vi "xiLIB - GPIO_Editor.vi"(8 "error in (no error)":errorcluster, 11 "xiCam In":refnum<k24>) -> (0 "error out":errorcluster)   [LabVIEW 2018]
doc: "Dialog based GPIO editor."
uses:
  xiCam/PRM/GPI_MODE/GPI_MODE.ctl
  xiCam/PRM/GPO_MODE/GPO_MODE.ctl
  D:/codes labview/VisionLibrariesXimea/xiLib/xiLIB_64bit/xiLIB/xiCamLib/API/x64/xiApi.NETX64.dll
  API/x64/xiApi.NETX64.dll
  xiCam/PRM/PRM/PRM_v2.ctl
panel:
  in  "GPO_MODE":T1
  in  "GPO_SELECTOR":u16(ring) items=["GPO 1"=1]
  in  "GPI_MODE":T2
  in  "GPI_SELECTOR":u16(ring) items=["GPI 1"=1]
  # "GPI/O Settings"
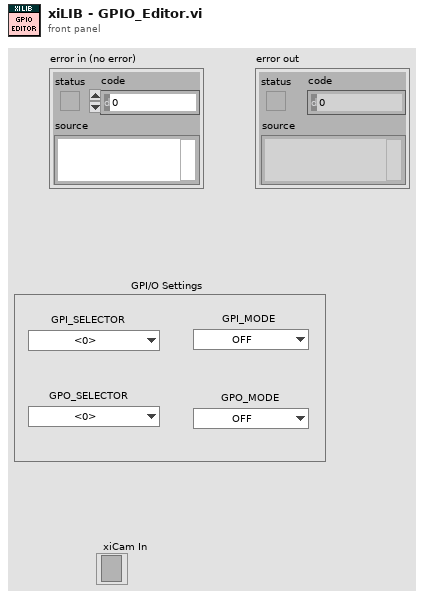
[diagram p1: front panel]
types:
  T1 = typedef "GPO_MODE.ctl" = enum16{"OFF", "ON", "FRAME_ACTIVE", "FRAME_ACTIVE_NEG", "EXPOSURE_ACTIVE", "EXPOSURE_ACTIVE_NEG"}
  T2 = typedef "GPI_MODE.ctl" = enum16{"OFF", "TRIGGER", "EXT_EVENT"}
  T3 = typedef "PRM_v2.ctl" = enum16{"ACQ_BUFFER_SIZE", "ACQ_FRAME_BURST_COUNT", "ACQ_TIMING_MODE", "ACQ_TRANSPORT_BUFFER_SIZE", "AE_MAX_LIMIT", "AEAG", "AEAG_LEVEL", "API_VERSION", "AG_MAX_LIMIT", "APPLY_CMS", "AUTO_BANDWIDTH_CALCULATION", "AUTO_WB", "AVAILABLE_BANDWIDTH", "AVAILABLE_BANDWIDTH_MAX", "AVAILABLE_BANDWIDTH_MIN", "BPC", "BUFFER_POLICY", "BUFFERS_QUEUE_SIZE", "CC_MATRIX_00", "CC_MATRIX_01", "CC_MATRIX_02", "CC_MATRIX_03", "CC_MATRIX_10", "CC_MATRIX_11", "CC_MATRIX_12", "CC_MATRIX_13", "CC_MATRIX_20", "CC_MATRIX_21", "CC_MATRIX_22", "CC_MATRIX_23", "CC_MATRIX_30", "CC_MATRIX_31", "CC_MATRIX_32", "CC_MATRIX_33", "CHIP_TEMP", "CMS", "COLOR_FILTER_ARRAY", "COOLING", "DEBOUNCE_EN", "DEBOUNCE_POL", "DEBOUNCE_T0", "DEBOUNCE_T1", "DEBUG_LEVEL", "DEFAULT_CC_MATRIX", "DEVICE_INSTANCE_PATH", "DEVICE_MODEL_ID", "DEVICE_NAME", "DEVICE_SN", "DEVICE_TYPE", "DEVICE_USER_ID", "DOWNSAMPLING", "DOWNSAMPLING_MAX", "DOWNSAMPLING_MIN", "DOWNSAMPLING_TYPE", "DRV_VERSION", "EXP_PRIORITY", "EXPOSURE", "EXPOSURE_DIRECT_UPDATE", "EXPOSURE_MAX", "EXPOSURE_MIN", "FFS_FILE_NAME", "FPGA1_VERSION", "FRAMERATE", "FRAMERATE_MAX", "FRAMERATE_MIN", "FREE_FFS_SIZE", "GAIN", "GAIN_DIRECT_UPDATE", "GAIN_MAX", "GAIN_MIN", "GAMMAC", "GAMMAY", "GPI_LEVEL", "GPI_MODE", "GPI_SELECTOR", "GPI_SELECTOR_MAX", "GPI_SELECTOR_MIN", "GPO_MODE", "GPO_SELECTOR", "GPO_SELECTOR_MAX", "GPO_SELECTOR_MIN", "HDR", "HDR_T1", "HDR_T2", "HEIGHT", "HEIGHT_MAX", "HEIGHT_MIN", "HOUSE_TEMP", "IMAGE_DATA_FORMAT", "IMAGE_IS_COLOR", "INPUT_CMS_PROFILE", "IS_COOLED", "IS_DEVICE_EXIST", "KNEEPOINT1", "KNEEPOINT2", "LED_MODE", "LED_SELECTOR", "LED_SELECTOR_MAX", "LED_SELECTOR_MIN", "LIMIT_BANDWIDTH", "LIMIT_BANDWIDTH_MAX", "LIMIT_BANDWIDTH_MIN", "LUT_EN", "LUT_INDEX", "LUT_INDEX_MAX", "LUT_INDEX_MIN", "LUT_VALUE", "LUT_VALUE_MAX", "LUT_VALUE_MIN", "MANUAL_WB", "MCU1_VERSION", "MCU2_VERSION", "OFFSET_X", "OFFSET_X_MAX", "OFFSET_X_MIN", "OFFSET_Y", "OFFSET_Y_MAX", "OFFSET_Y_MIN", "OUTPUT_CMS_PROFILE", "OUTPUT_DATA_BIT_DEPTH", "OUTPUT_DATA_PACKING", "READ_FILE_FFS", "RECENT_FRAME", "SENSOR_DATA_BIT_DEPTH", "SENSOR_MODE", "SENSOR_TAPS", "SHARPNESS", "SHUTTER_TYPE", "TARGET_TEMP", "TRG_DELAY", "TRG_SELECTOR", "TRG_SOFTWARE", "TRG_SOURCE", "USED_FFS_SIZE", "WB_KB", "WB_KG", "WB_KR", "WIDTH", "WIDTH_MAX", "WIDTH_MIN", "WRITE_FILE_FFS", "ACQ_BUFFER_SIZE_UNIT", "ACQ_TRANSPORT_BUFFER_COMMIT", "AEAG_ROI_HEIGHT", "AEAG_ROI_OFFSET_X", "AEAG_ROU_OFFSET_Y", "AEAG_ROI_WIDTH", "API_CONTEXT_LIST", "BINNING_HORIZONTAL", "BINNING_SELECTOR", "BINNING_VERTICAL", "COLUMN_FPN_CORRECTION", "COUNTER_SELECTOR", "COUNTER_VALUE", "DECIMATION_HORIZONTAL", "DECIMATION_SELECTOR", "DECIMATION_VERTICAL", "DEVICE_ID", "DEVICE_LOCATION_PATH", "DEVICE_MANIFEST", "DEVICE_RESET", "DEVICE_SENS_SN", "EXPOSURE_BURST_COUNT", "FFS_ACCESS_KEY", "GAIN_SELECTOR", "HW_REVISION", "IMAGE_BLACK_LEVEL", "IMAGE_DATA_BIT_DEPTH", "IMAGE_DATA_FORMAT_RGB32_ALPHA", "IMAGE_PAYLOAD_SIZE", "LENS_APERTURE_VALUE", "LENS_FEATURE", "LENS_FEATURE_SELECTOR", "LENS_FOCAL_LENGTH", "LENS_FOCUS_DISTANCE", "LENS_FOCUS_MOVE", "LENS_FOCUS_MOVEMENT_VALUE", "LENS_MODE", "OUTPUT_DATA_PACKING_TYPE", "SENSOR_CLOCK_FREQ_HZ", "SENSOR_CLOCK_FREQ_INDEX", "SENSOR_FEATURE_SELECTOR", "SENSOR_FEATURE_VALUE", "SENSOR_OUTPUT_CHANNEL_COUNT", "TRANSPORT_PIXEL_FORMAT", "TS_RST_MODE", "TS_RST_SOURCE"}
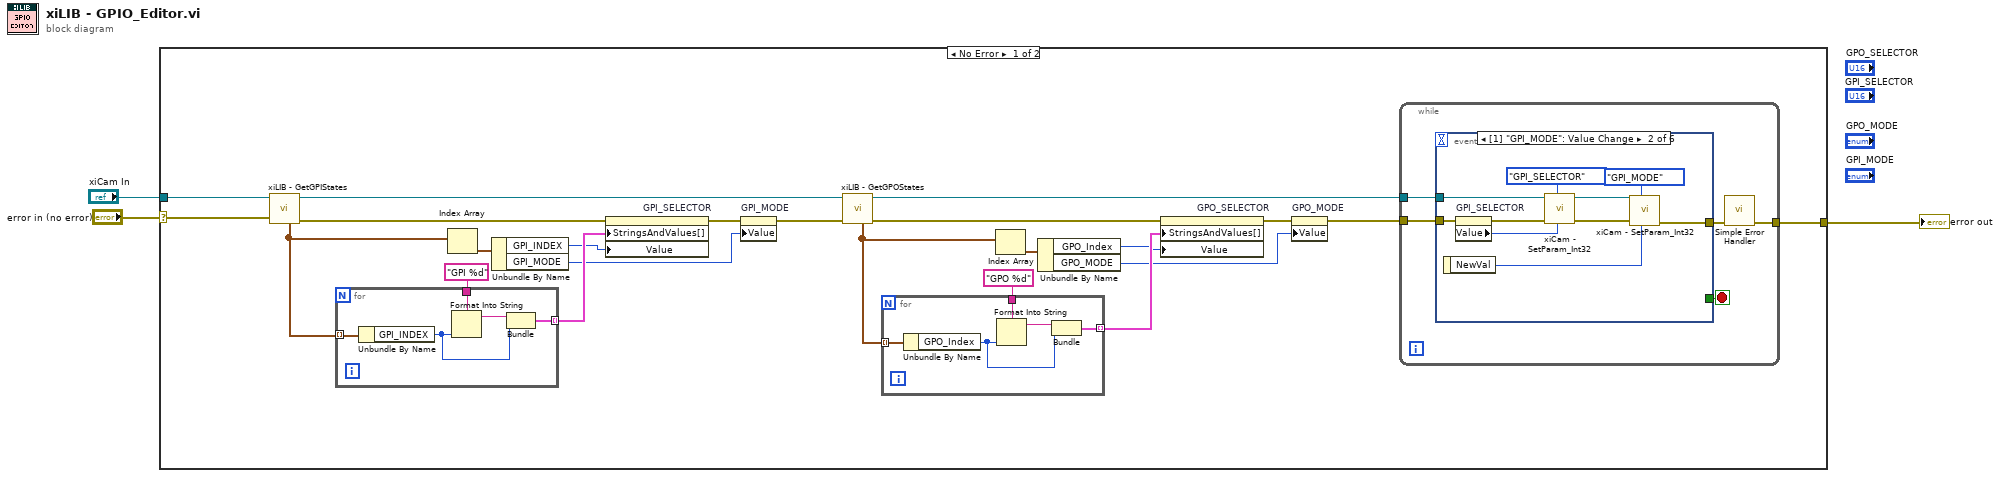
[diagram p0: block diagram]
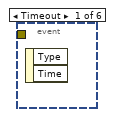
[diagram p2: hidden frame]
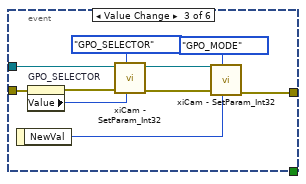
[diagram p3: hidden frame]
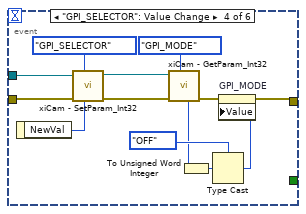
[diagram p4: hidden frame]
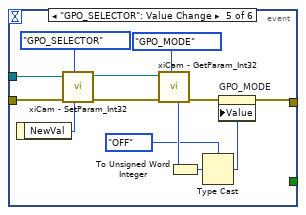
[diagram p5: hidden frame]
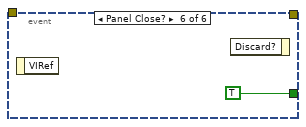
[diagram p6: hidden frame]
diagram:
  n1 = case shown="No Error" "error in (no error)" {
    selector: "error in (no error)" -> [w26 w89]
    tunnel: [w18 w89] -> w2
    tunnel: "xiCam In" -> [w4 _]
    frame No Error {
      n2 = call "xiLIB - GetGPIStates.vi"("error in (no error)"=w26, "xiCam In"=w4) -> ("error out"=w25:errorcluster, "xiCam Out"=w23:refnum<k24>, "GPI_States[] - NUM"=w16:cluster{"GPI_INDEX":i32, "GPI_MODE":T2}[])  [unwired: 6 in, 1 out]
      n3 = for {
        tunnel: w16 -> [w88] mode=indexing
        tunnel: [w85] -> w17 mode=indexing
        tunnel: "GPI %d" ("format string") -> [w84]
        n4 = Unbundle By Name(w88) -> ("GPI_INDEX"=w86:i32)
        n5 = Format Into String(format string=w84, w86) -> (resulting string=w87:string)  [unwired: 2 in, 1 out]
        n6 = Bundle(w87, "GPI_INDEX"=w86) -> (w85:cluster{string, "GPI_INDEX":i32})  [unwired: 1 in]
      }
      n7 = Index Array(array=w16) -> (element=w15:cluster{"GPI_INDEX":i32, "GPI_MODE":T2})  [unwired: 1 in]
      n8 = Unbundle By Name(w15) -> ("GPI_INDEX"=w14:i32, "GPI_MODE"=w11:T2)
      n9 = property on="GPI_SELECTOR" class="Ring (strict)"(error in=w25, "StringsAndValues[]"=w17, "Value"=w14) -> (error out=w13:errorcluster)  [unwired: 1 in, 1 out]
      n10 = property on="GPI_MODE" class="Enum (strict)"(error in=w13, "Value"=w11) -> (error out=w12:errorcluster)  [unwired: 1 in, 1 out]
      n11 = call "xiLIB - GetGPOStates.vi"("error in (no error)"=w12, "xiCam In"=w23) -> ("error out"=w21:errorcluster, "xiCam Out"=w19:refnum<k24>, "GPO_States[] - NUM"=w9:cluster{"GPO_Index":i32, "GPO_MODE":T1}[])  [unwired: 6 in, 1 out]
      n12 = for {
        tunnel: w9 -> [w83] mode=indexing
        tunnel: [w80] -> w20 mode=indexing
        tunnel: "GPO %d" ("format string") -> [w79]
        n13 = Unbundle By Name(w83) -> ("GPO_Index"=w81:i32)
        n14 = Format Into String(format string=w79, w81) -> (resulting string=w82:string)  [unwired: 2 in, 1 out]
        n15 = Bundle(w82, "GPO_Index"=w81) -> (w80:cluster{string, "GPO_Index":i32})  [unwired: 1 in]
      }
      n16 = Index Array(array=w9) -> (element=w10:cluster{"GPO_Index":i32, "GPO_MODE":T1})  [unwired: 1 in]
      n17 = Unbundle By Name(w10) -> ("GPO_Index"=w8:i32, "GPO_MODE"=w5:T1)
      n18 = property on="GPO_SELECTOR" class="Ring (strict)"(error in=w21, "StringsAndValues[]"=w20, "Value"=w8) -> (error out=w7:errorcluster)  [unwired: 1 in, 1 out]
      n19 = property on="GPO_MODE" class="Enum (strict)"(error in=w7, "Value"=w5) -> (error out=w6:errorcluster)  [unwired: 1 in, 1 out]
      n20 = while {
        tunnel: w6 -> [w29]
        tunnel: w19 -> [w30]
        tunnel: [w27] -> w18
        stop <- w31 stop-if-true
        n21 = event shown="[1] \"GPI_MODE\": Value Change" {
          selector: _ -> [_ _ _ _ _ _]
          dyn-events: _ -> [_ _ _ _ _ _]
          timeout: _ -> [_ _ _ _ _ _]
          tunnel: [_ _ _ _ _ TRUE] -> w31
          tunnel: w30 -> [_ w38 w50 w60 w75 _]
          tunnel: w29 -> [_ w39 w44 w59 w74 _]
          tunnel: [_ w32 w45 w54 w70 _] -> w28
          event Timeout {
            n22 = event-data() -> ()  [unwired: 1 in, 2 out]
          }
          event Value Change {
            n23 = event-data() -> ("NewVal"=w33:T2)  [unwired: 1 in]
            n24 = property on="GPI_SELECTOR" class="Ring (strict)"(error in=w39) -> (error out=w40:errorcluster, "Value"=w37:u16)  [unwired: 1 in, 1 out]
            n25 = call "xiCam - SetParam_Int32.vi"("Int32_Value"=w37, "PRM"=PRM_v2."GPI_SELECTOR", "error in (no error)"=w40, "xiCam In"=w38) -> ("error out"=w35:errorcluster, "xiCam Out"=w36:refnum<k24>)  [unwired: 6 in]
            n26 = call "xiCam - SetParam_Int32.vi"("Int32_Value"=w33, "PRM"=PRM_v2."GPI_MODE", "error in (no error)"=w35, "xiCam In"=w36) -> ("error out"=w32:errorcluster)  [unwired: 6 in, 1 out]
          }
          event Value Change {
            n27 = event-data() -> ("NewVal"=w46:T1)  [unwired: 1 in]
            n28 = property on="GPO_SELECTOR" class="Ring (strict)"(error in=w44) -> (error out=w43:errorcluster, "Value"=w42:u16)  [unwired: 1 in, 1 out]
            n29 = call "xiCam - SetParam_Int32.vi"("Int32_Value"=w42, "PRM"=PRM_v2."GPO_SELECTOR", "error in (no error)"=w43, "xiCam In"=w50) -> ("error out"=w48:errorcluster, "xiCam Out"=w49:refnum<k24>)  [unwired: 6 in]
            n30 = call "xiCam - SetParam_Int32.vi"("Int32_Value"=w46, "PRM"=PRM_v2."GPO_MODE", "error in (no error)"=w48, "xiCam In"=w49) -> ("error out"=w45:errorcluster)  [unwired: 6 in, 1 out]
          }
          event "GPI_SELECTOR": Value Change {
            n31 = event-data() -> ("NewVal"=w58:u16)  [unwired: 1 in]
            n32 = call "xiCam - SetParam_Int32.vi"("Int32_Value"=w58, "PRM"=PRM_v2."GPI_SELECTOR", "error in (no error)"=w59, "xiCam In"=w60) -> ("error out"=w64:errorcluster, "xiCam Out"=w63:refnum<k24>)  [unwired: 6 in]
            n33 = call "xiCam - GetParam_Int32.vi"("PRM"=PRM_v2."GPI_MODE", "error in (no error)"=w64, "xiCam In"=w63) -> ("error out"=w55:errorcluster, "Int32_Value"=w56:i32)  [unwired: 6 in, 1 out]
            n34 = To Unsigned Word Integer(number=w56) -> (unsigned 16bit integer=w52:u16)
            n35 = Type Cast(type=GPI_MODE."OFF" ("GPI_MODE"), x=w52) -> (*(type *) &x=w53:T2)
            n36 = property on="GPI_MODE" class="Enum (strict)"(error in=w55, "Value"=w53) -> (error out=w54:errorcluster)  [unwired: 1 in, 1 out]
          }
          event "GPO_SELECTOR": Value Change {
            n37 = event-data() -> ("NewVal"=w73:u16)  [unwired: 1 in]
            n38 = call "xiCam - SetParam_Int32.vi"("Int32_Value"=w73, "PRM"=PRM_v2."GPO_SELECTOR", "error in (no error)"=w74, "xiCam In"=w75) -> ("error out"=w77:errorcluster, "xiCam Out"=w76:refnum<k24>)  [unwired: 6 in]
            n39 = call "xiCam - GetParam_Int32.vi"("PRM"=PRM_v2."GPO_MODE", "error in (no error)"=w77, "xiCam In"=w76) -> ("error out"=w71:errorcluster, "Int32_Value"=w72:i32)  [unwired: 6 in, 1 out]
            n40 = To Unsigned Word Integer(number=w72) -> (unsigned 16bit integer=w67:u16)
            n41 = Type Cast(type=GPO_MODE."OFF" ("GPO_MODE"), x=w67) -> (*(type *) &x=w69:T1)
            n42 = property on="GPO_MODE" class="Enum (strict)"(error in=w71, "Value"=w69) -> (error out=w70:errorcluster)  [unwired: 1 in, 1 out]
          }
          event Panel Close? {
            n43 = event-data() -> ()  [unwired: 1 in, 1 out]
            n44 = event-data() -> ()  [unwired: 2 in, 1 out]
          }
        }
        n45 = call <vilib>:"Simple Error Handler.vi"("error in (no error)"=w28) -> ("error out"=w27:errorcluster)  [unwired: 4 in, 4 out]
      }
    }
    frame Error {
    }
  }
  "error out" <- w2
